vi "TCP Communicator - Active2.vi"() -> ()   [LabVIEW 2019]
panel:
  out "BL_Receive":T1 {"ControlScheme"."Time" format="%<%Y-%m-%d %H:%M:%S>T"; "ControllerConfig"."Time" format="%<%Y-%m-%d %H:%M:%S>T"; "BalancingMotor-All"."BalancingMotor-00"."Time" format="%<%Y-%m-%d %H:%M:%S>T"; "BalancingMotor-All"."BalancingMotor-01"."Time" format="%<%Y-%m-%d %H:%M:%S>T"; "BalancingMotor-All"."BalancingMotor-02"."Time" format="%<%Y-%m-%d %H:%M:%S>T"; "BalancingMotor-All"."BalancingMotor-03"."Time" format="%<%Y-%m-%d %H:%M:%S>T"}
  in  "BL_Send":T1 {"ControlScheme"."Time" format="%<%Y-%m-%d %H:%M:%S>T"; "ControllerConfig"."Time" format="%<%Y-%m-%d %H:%M:%S>T"; "BalancingMotor-All"."BalancingMotor-00"."Time" format="%<%Y-%m-%d %H:%M:%S>T"; "BalancingMotor-All"."BalancingMotor-01"."Time" format="%<%Y-%m-%d %H:%M:%S>T"; "BalancingMotor-All"."BalancingMotor-02"."Time" format="%<%Y-%m-%d %H:%M:%S>T"; "BalancingMotor-All"."BalancingMotor-03"."Time" format="%<%Y-%m-%d %H:%M:%S>T"}
  out "BL_Send2":T1 {"ControlScheme"."Time" format="%<%Y-%m-%d %H:%M:%S>T"; "ControllerConfig"."Time" format="%<%Y-%m-%d %H:%M:%S>T"; "BalancingMotor-All"."BalancingMotor-00"."Time" format="%<%Y-%m-%d %H:%M:%S>T"; "BalancingMotor-All"."BalancingMotor-01"."Time" format="%<%Y-%m-%d %H:%M:%S>T"; "BalancingMotor-All"."BalancingMotor-02"."Time" format="%<%Y-%m-%d %H:%M:%S>T"; "BalancingMotor-All"."BalancingMotor-03"."Time" format="%<%Y-%m-%d %H:%M:%S>T"}
  in  "stop":bool
  in  "Port":u16=6343
  in  "Machine":string="192.168.150.9"
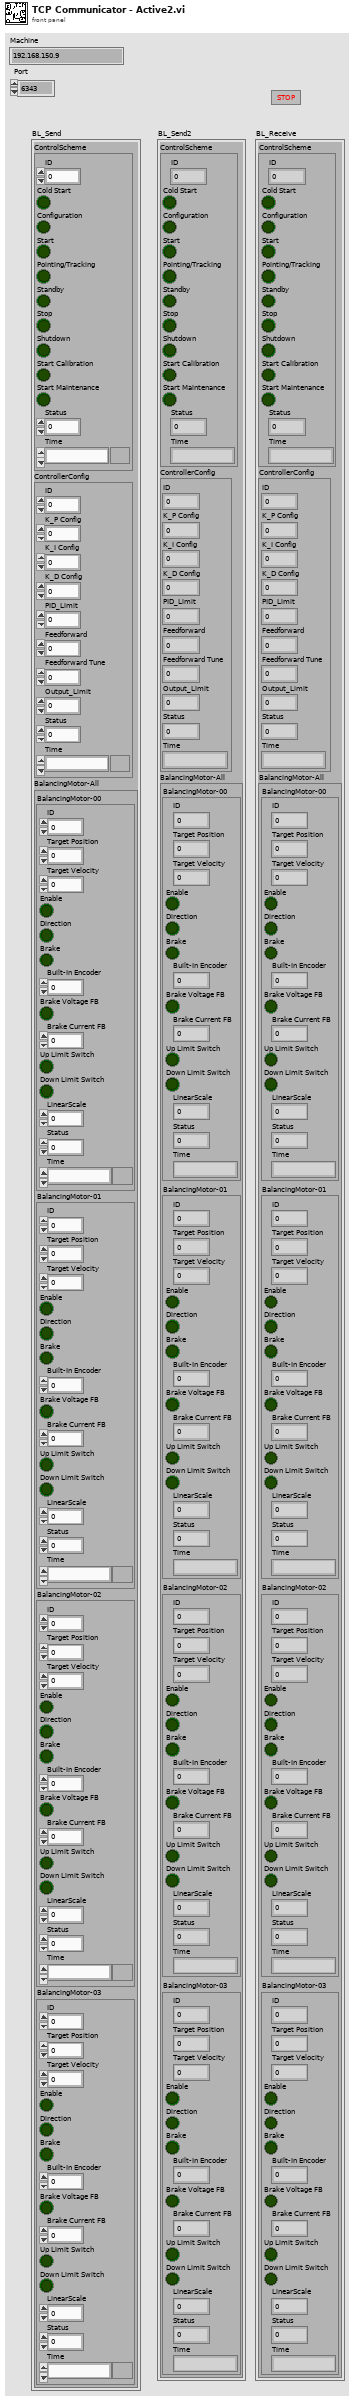
[diagram p1: front panel]
types:
  T1 = cluster{"ControlScheme":cluster{"ID":i32, "Cold Start":bool, "Configuration":bool, "Start":bool, "Pointing/Tracking":bool, "Standby":bool, "Stop":bool, "Shutdown":bool, "Start Calibration":bool, "Start Maintenance":bool, "Status":i16, "Time ":timestamp}, "ControllerConfig":cluster{"ID":i32, "K_P Config":u64, "K_I Config":u64, "K_D Config":u64, "PID_Limit":u64, "Feedforward":u64, "Feedforward Tune":u64, "Output_Limit":u64, "Status":i16, "Time ":timestamp}, "BalancingMotor-All":cluster{"BalancingMotor-00":cluster{"ID":i32, "Target Position":u64, "Target Velocity":u64, "Enable":bool, "Direction":bool, "Brake":bool, "Built-In Encoder":u64, "Brake Voltage FB":bool, "Brake Current FB":u64, "Up Limit Switch":bool, "Down Limit Switch":bool, "LinearScale":u64, "Status":i16, "Time ":timestamp}, "BalancingMotor-01":cluster{"ID":i32, "Target Position":u64, "Target Velocity":u64, "Enable":bool, "Direction":bool, "Brake":bool, "Built-In Encoder":u64, "Brake Voltage FB":bool, "Brake Current FB":u64, "Up Limit Switch":bool, "Down Limit Switch":bool, "LinearScale":u64, "Status":i16, "Time ":timestamp}, "BalancingMotor-02":cluster{"ID":i32, "Target Position":u64, "Target Velocity":u64, "Enable":bool, "Direction":bool, "Brake":bool, "Built-In Encoder":u64, "Brake Voltage FB":bool, "Brake Current FB":u64, "Up Limit Switch":bool, "Down Limit Switch":bool, "LinearScale":u64, "Status":i16, "Time ":timestamp}, "BalancingMotor-03":cluster{"ID":i32, "Target Position":u64, "Target Velocity":u64, "Enable":bool, "Direction":bool, "Brake":bool, "Built-In Encoder":u64, "Brake Voltage FB":bool, "Brake Current FB":u64, "Up Limit Switch":bool, "Down Limit Switch":bool, "LinearScale":u64, "Status":i16, "Time ":timestamp}}}
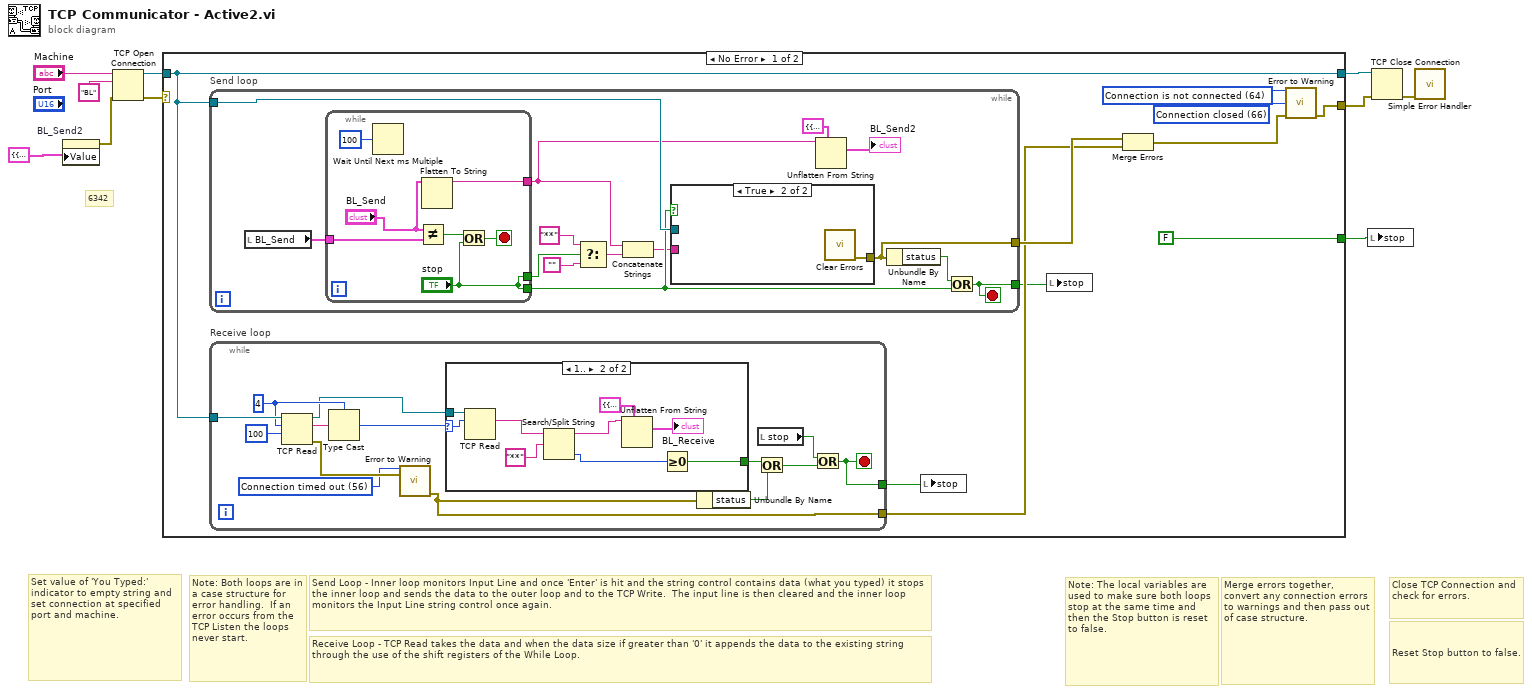
[diagram p0: block diagram]
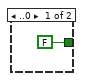
[diagram p2: hidden frame]
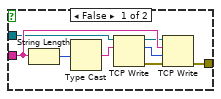
[diagram p3: hidden frame]
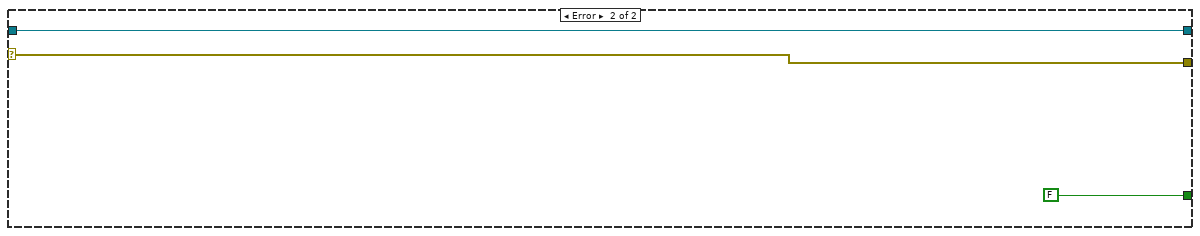
[diagram p4: hidden frame]
diagram:
  # "6342"
  # "Set value of 'You Typed:' indicator to empty string and set connection at specified port and machine."
  # "Send Loop - Inner loop monitors Input Line and once 'Enter' is hit and the string control contains data (what you typed) it stops the inner loop and sends the data to the outer loop and to the TCP Write.  The input line is then cleared and the inner loop monitors the Input Line string control once again."
  # "Receive Loop - TCP Read takes the data and when the data size if greater than '0' it appends the data to the existing string through the use of the shift registers of the While Loop."
  # "Note: The local variables are used to make sure both loops stop at the same time and then the Stop button is reset to false."
  # "Merge errors together, convert any connection errors to warnings and then pass out of case structure."
  # "Note: Both loops are in a case structure for error handling.  If an error occurs from the TCP Listen the loops never start."
  # "Close TCP Connection and check for errors."
  # "Reset Stop button to false."
  n1 = property on="BL_Send2" class="Clust (strict)"("Value"=T1 {"ControlScheme"={"ID"=0, "Cold Start"=FALSE, "Configuration"=FALSE, "Start"=FALSE, "Pointing/Tracking"=FALSE, "Standby"=FALSE, "Stop"=FALSE, "Shutdown"=FALSE, "Start Calibration"=FALSE, "Start Maintenance"=FALSE, "Status"=0, "Time "=timestamp(0 s since 1904-01-01)}, "ControllerConfig"={"ID"=0, "K_P Config"=0, "K_I Config"=0, "K_D Config"=0, "PID_Limit"=0, "Feedforward"=0, "Feedforward Tune"=0, "Output_Limit"=0, "Status"=0, "Time "=timestamp(0 s since 1904-01-01)}, "BalancingMotor-All"={"BalancingMotor-00"={"ID"=0, "Target Position"=0, "Target Velocity"=0, "Enable"=FALSE, "Direction"=FALSE, "Brake"=FALSE, "Built-In Encoder"=0, "Brake Voltage FB"=FALSE, "Brake Current FB"=0, "Up Limit Switch"=FALSE, "Down Limit Switch"=FALSE, "LinearScale"=0, "Status"=0, "Time "=timestamp(0 s since 1904-01-01)}, "BalancingMotor-01"={"ID"=0, "Target Position"=0, "Target Velocity"=0, "Enable"=FALSE, "Direction"=FALSE, "Brake"=FALSE, "Built-In Encoder"=0, "Brake Voltage FB"=FALSE, "Brake Current FB"=0, "Up Limit Switch"=FALSE, "Down Limit Switch"=FALSE, "LinearScale"=0, "Status"=0, "Time "=timestamp(0 s since 1904-01-01)}, "BalancingMotor-02"={"ID"=0, "Target Position"=0, "Target Velocity"=0, "Enable"=FALSE, "Direction"=FALSE, "Brake"=FALSE, "Built-In Encoder"=0, "Brake Voltage FB"=FALSE, "Brake Current FB"=0, "Up Limit Switch"=FALSE, "Down Limit Switch"=FALSE, "LinearScale"=0, "Status"=0, "Time "=timestamp(0 s since 1904-01-01)}, "BalancingMotor-03"={"ID"=0, "Target Position"=0, "Target Velocity"=0, "Enable"=FALSE, "Direction"=FALSE, "Brake"=FALSE, "Built-In Encoder"=0, "Brake Voltage FB"=FALSE, "Brake Current FB"=0, "Up Limit Switch"=FALSE, "Down Limit Switch"=FALSE, "LinearScale"=0, "Status"=0, "Time "=timestamp(0 s since 1904-01-01)}}} ("BL_Send")) -> (error out=w3:errorcluster)  [unwired: 2 in, 1 out]
  n2 = TCP Open Connection(address="Machine", remote port or service name="BL" ("service name"), error in (no error)=w3) -> (connection ID=w8:refnum<k5>, error out=w9:errorcluster)  [unwired: 2 in]
  n3 = case shown="No Error" w9 {
    selector: w9 -> [_ w76]
    tunnel: [w17 w76] -> w6
    tunnel: w8 -> [w11 w77]
    tunnel: [w11 w77] -> w7
    tunnel: [FALSE FALSE] -> w4
    frame No Error {
      w18 = 66 items=["No Error", "Argument Error", "Memory Full", "Out of Zone", "End of File", "File Already Open", "Generic File IO Error", "File Not Found", "File Permission Error", "Disk Full", "Duplicate Path", "Too Many Files Open", "Not Enabled", "Resource File Not Found", "Cannot Add Resource", "Resource Not Found", "Image Not Found", "Image Memory Error", "Pen Does Not Exist", "Config Bad Type", "Config Token Not Found", "Config Parse Error", "Config Memory Error", "Bad External Code Format", "Bad External Code Offset", "External Code Not Present", "Null Window", "Destroy Window Mixup", "Null Menu", "Print Aborted", "Bad Print Record", "Print Driver Error", "Windows Error During Print", "Memory Error During Print", "Print Dialog Error", "Generic Print Error", "Invalid Device Refnum", "Device Not Found", "Device Parameter Error", "Device Unit Error", "Can't Open Device", "Device Call Aborted", "Generic Error", "Cancelled By User", "Object ID Too Low", "Object ID Too High", "Object Not In Heap", "Unknown Heap", "Bad DefProc ID", "DefProc Not In Table", "Message Out Of Range", "Null Method", "Unknown Message", "Manager Call Not Supported", "Bad address", "Connection In progress", "Connection timed out", "Connection is already in progress", "Network attribute not supported", "Network error", "Address in use", "System out of memory", "Connection aborted", "Connection refused", "Connection is not connected", "Connection is already connected", "Connection closed", "Initialize error (interapplication manager)", "Bad occurrence", "Wait on unbound occurrence handler", "Occurrence queue overflow", "Bad path", "Semaphore not signaled", "Unrecognized type (interapplication manager)"] ("3rd Error to Convert")
      w19 = 64 items=["No Error", "Argument Error", "Memory Full", "Out of Zone", "End of File", "File Already Open", "Generic File IO Error", "File Not Found", "File Permission Error", "Disk Full", "Duplicate Path", "Too Many Files Open", "Not Enabled", "Resource File Not Found", "Cannot Add Resource", "Resource Not Found", "Image Not Found", "Image Memory Error", "Pen Does Not Exist", "Config Bad Type", "Config Token Not Found", "Config Parse Error", "Config Memory Error", "Bad External Code Format", "Bad External Code Offset", "External Code Not Present", "Null Window", "Destroy Window Mixup", "Null Menu", "Print Aborted", "Bad Print Record", "Print Driver Error", "Windows Error During Print", "Memory Error During Print", "Print Dialog Error", "Generic Print Error", "Invalid Device Refnum", "Device Not Found", "Device Parameter Error", "Device Unit Error", "Can't Open Device", "Device Call Aborted", "Generic Error", "Cancelled By User", "Object ID Too Low", "Object ID Too High", "Object Not In Heap", "Unknown Heap", "Bad DefProc ID", "DefProc Not In Table", "Message Out Of Range", "Null Method", "Unknown Message", "Manager Call Not Supported", "Bad address", "Connection In progress", "Connection timed out", "Connection is already in progress", "Network attribute not supported", "Network error", "Address in use", "System out of memory", "Connection aborted", "Connection refused", "Connection is not connected", "Connection is already connected", "Connection closed", "Initialize error (interapplication manager)", "Bad occurrence", "Wait on unbound occurrence handler", "Occurrence queue overflow", "Bad path", "Semaphore not signaled", "Unrecognized type (interapplication manager)"] ("1st Error to Convert")
      n4 = while "Send loop" {
        tunnel: w11 -> [w57]
        tunnel: [w58] -> w12
        tunnel: [w53] -> w15
        stop <- w58 stop-if-true
        n5 = local read "BL_Send"() -> (w50:T1)
        n6 = while {
          tunnel: ["stop"] -> w55
          tunnel: ["stop"] -> w51
          tunnel: [w60] -> w49
          tunnel: w50 -> [w62]
          stop <- w63 stop-if-true
          n7 = Wait Until Next ms Multiple(millisecond multiple=u32 100) -> ()  [unwired: 1 out]
          n8 = Not Equal?(x="BL_Send", y=w62) -> (x != y?=w64:bool)
          n9 = Flatten To String(anything="BL_Send") -> (data string=w60:string)  [unwired: 3 in, 2 out]
          n10 = Or(x=w64, y="stop") -> (x .or. y?=w63:bool)
        }
        n11 = Select(t="**", s=w55, f="") -> (s? t:f=w48:string)
        n12 = Concatenate Strings(w49, w48) -> (w47:string)
        n13 = case shown="True" w51 {
          tunnel: w47 -> [w70 _]
          tunnel: [w73 w74] -> w53
          tunnel: w57 -> [w67 _]
          frame False {
            n14 = String Length(string=w70) -> (length=w69:i32)
            n15 = Type Cast(x=w69) -> (*(type *) &x=w68:string)  [unwired: 1 in]
            n16 = TCP Write(connection ID=w67, data in=w68) -> (connection ID out=w66:refnum<k5>, bytes written=w71:i32, error out=w72:errorcluster)  [unwired: 2 in]
            n17 = TCP Write(connection ID=w66, data in=w70, error in (no error)=w72, 9:w71) -> (error out=w73:errorcluster)  [unwired: 2 out]
          }
          frame True {
            n18 = call <vilib>:"Clear Errors.vi"() -> ("error out"=w74:errorcluster)  [unwired: 6 in, 1 out]
          }
        }
        n19 = Unflatten From String(type=T1 {"ControlScheme"={"ID"=0, "Cold Start"=FALSE, "Configuration"=FALSE, "Start"=FALSE, "Pointing/Tracking"=FALSE, "Standby"=FALSE, "Stop"=FALSE, "Shutdown"=FALSE, "Start Calibration"=FALSE, "Start Maintenance"=FALSE, "Status"=0, "Time "=timestamp(0 s since 1904-01-01)}, "ControllerConfig"={"ID"=0, "K_P Config"=0, "K_I Config"=0, "K_D Config"=0, "PID_Limit"=0, "Feedforward"=0, "Feedforward Tune"=0, "Output_Limit"=0, "Status"=0, "Time "=timestamp(0 s since 1904-01-01)}, "BalancingMotor-All"={"BalancingMotor-00"={"ID"=0, "Target Position"=0, "Target Velocity"=0, "Enable"=FALSE, "Direction"=FALSE, "Brake"=FALSE, "Built-In Encoder"=0, "Brake Voltage FB"=FALSE, "Brake Current FB"=0, "Up Limit Switch"=FALSE, "Down Limit Switch"=FALSE, "LinearScale"=0, "Status"=0, "Time "=timestamp(0 s since 1904-01-01)}, "BalancingMotor-01"={"ID"=0, "Target Position"=0, "Target Velocity"=0, "Enable"=FALSE, "Direction"=FALSE, "Brake"=FALSE, "Built-In Encoder"=0, "Brake Voltage FB"=FALSE, "Brake Current FB"=0, "Up Limit Switch"=FALSE, "Down Limit Switch"=FALSE, "LinearScale"=0, "Status"=0, "Time "=timestamp(0 s since 1904-01-01)}, "BalancingMotor-02"={"ID"=0, "Target Position"=0, "Target Velocity"=0, "Enable"=FALSE, "Direction"=FALSE, "Brake"=FALSE, "Built-In Encoder"=0, "Brake Voltage FB"=FALSE, "Brake Current FB"=0, "Up Limit Switch"=FALSE, "Down Limit Switch"=FALSE, "LinearScale"=0, "Status"=0, "Time "=timestamp(0 s since 1904-01-01)}, "BalancingMotor-03"={"ID"=0, "Target Position"=0, "Target Velocity"=0, "Enable"=FALSE, "Direction"=FALSE, "Brake"=FALSE, "Built-In Encoder"=0, "Brake Voltage FB"=FALSE, "Brake Current FB"=0, "Up Limit Switch"=FALSE, "Down Limit Switch"=FALSE, "LinearScale"=0, "Status"=0, "Time "=timestamp(0 s since 1904-01-01)}}} ("BL_Send"), binary string=w49) -> (value=→"BL_Send2":T1)  [unwired: 3 in, 2 out]
        n20 = Unbundle By Name(w53) -> ("status"=w52:bool)
        n21 = Or(x=w52, y=w51) -> (x .or. y?=w58:bool)
      }
      n22 = while "Receive loop" {
        tunnel: [w33] -> w14
        tunnel: [w28] -> w13
        tunnel: w11 -> [w34]
        stop <- w33 stop-if-true
        w23 = 4
        w29 = 56 items=["No Error", "Argument Error", "Memory Full", "Out of Zone", "End of File", "File Already Open", "Generic File IO Error", "File Not Found", "File Permission Error", "Disk Full", "Duplicate Path", "Too Many Files Open", "Not Enabled", "Resource File Not Found", "Cannot Add Resource", "Resource Not Found", "Image Not Found", "Image Memory Error", "Pen Does Not Exist", "Config Bad Type", "Config Token Not Found", "Config Parse Error", "Config Memory Error", "Bad External Code Format", "Bad External Code Offset", "External Code Not Present", "Null Window", "Destroy Window Mixup", "Null Menu", "Print Aborted", "Bad Print Record", "Print Driver Error", "Windows Error During Print", "Memory Error During Print", "Print Dialog Error", "Generic Print Error", "Invalid Device Refnum", "Device Not Found", "Device Parameter Error", "Device Unit Error", "Can't Open Device", "Device Call Aborted", "Generic Error", "Cancelled By User", "Object ID Too Low", "Object ID Too High", "Object Not In Heap", "Unknown Heap", "Bad DefProc ID", "DefProc Not In Table", "Message Out Of Range", "Null Method", "Unknown Message", "Manager Call Not Supported", "Bad address", "Connection In progress", "Connection timed out", "Connection is already in progress", "Network attribute not supported", "Network error", "Address in use", "System out of memory", "Connection aborted", "Connection refused", "Connection is not connected", "Connection is already connected", "Connection closed", "Initialize error (interapplication manager)", "Bad occurrence", "Wait on unbound occurrence handler", "Occurrence queue overflow", "Bad path", "Semaphore not signaled", "Unrecognized type (interapplication manager)"] ("1st Error to Convert")
        n23 = TCP Read(connection ID=w34, bytes to read=w23, 9:100) -> (connection ID out=w21:refnum<k5>, data out=w24:string, error out=w30:errorcluster)  [unwired: 2 in]
        n24 = Type Cast(type=w23, x=w24) -> (*(type *) &x=w22:i32)
        n25 = call <vilib>:"Error to Warning.vi"("1st Error to Convert"=w29, "error in"=w30) -> ("warning out"=w28:errorcluster)  [unwired: 13 in]
        n26 = case shown="1.." w22 {
          selector: w22 -> [_ w44]
          tunnel: [FALSE w40] -> w32
          tunnel: w21 -> [_ w43]
          frame ..0 {
          }
          frame 1.. {
            n27 = TCP Read(connection ID=w43, bytes to read=w44) -> (data out=w37:string)  [unwired: 3 in, 2 out]
            n28 = Search/Split String(string=w37, search string/char (-)="**") -> (substring before match=w36:string, offset of match=w42:i32)  [unwired: 1 in, 1 out]
            n29 = Unflatten From String(type=T1 {"ControlScheme"={"ID"=0, "Cold Start"=FALSE, "Configuration"=FALSE, "Start"=FALSE, "Pointing/Tracking"=FALSE, "Standby"=FALSE, "Stop"=FALSE, "Shutdown"=FALSE, "Start Calibration"=FALSE, "Start Maintenance"=FALSE, "Status"=0, "Time "=timestamp(0 s since 1904-01-01)}, "ControllerConfig"={"ID"=0, "K_P Config"=0, "K_I Config"=0, "K_D Config"=0, "PID_Limit"=0, "Feedforward"=0, "Feedforward Tune"=0, "Output_Limit"=0, "Status"=0, "Time "=timestamp(0 s since 1904-01-01)}, "BalancingMotor-All"={"BalancingMotor-00"={"ID"=0, "Target Position"=0, "Target Velocity"=0, "Enable"=FALSE, "Direction"=FALSE, "Brake"=FALSE, "Built-In Encoder"=0, "Brake Voltage FB"=FALSE, "Brake Current FB"=0, "Up Limit Switch"=FALSE, "Down Limit Switch"=FALSE, "LinearScale"=0, "Status"=0, "Time "=timestamp(0 s since 1904-01-01)}, "BalancingMotor-01"={"ID"=0, "Target Position"=0, "Target Velocity"=0, "Enable"=FALSE, "Direction"=FALSE, "Brake"=FALSE, "Built-In Encoder"=0, "Brake Voltage FB"=FALSE, "Brake Current FB"=0, "Up Limit Switch"=FALSE, "Down Limit Switch"=FALSE, "LinearScale"=0, "Status"=0, "Time "=timestamp(0 s since 1904-01-01)}, "BalancingMotor-02"={"ID"=0, "Target Position"=0, "Target Velocity"=0, "Enable"=FALSE, "Direction"=FALSE, "Brake"=FALSE, "Built-In Encoder"=0, "Brake Voltage FB"=FALSE, "Brake Current FB"=0, "Up Limit Switch"=FALSE, "Down Limit Switch"=FALSE, "LinearScale"=0, "Status"=0, "Time "=timestamp(0 s since 1904-01-01)}, "BalancingMotor-03"={"ID"=0, "Target Position"=0, "Target Velocity"=0, "Enable"=FALSE, "Direction"=FALSE, "Brake"=FALSE, "Built-In Encoder"=0, "Brake Voltage FB"=FALSE, "Brake Current FB"=0, "Up Limit Switch"=FALSE, "Down Limit Switch"=FALSE, "LinearScale"=0, "Status"=0, "Time "=timestamp(0 s since 1904-01-01)}}} ("BL_Send"), binary string=w36) -> (value=→"BL_Receive":T1)  [unwired: 3 in, 2 out]
            n30 = Greater Or Equal To 0?(x=w42) -> (x >= 0?=w40:bool)
          }
        }
        n31 = Unbundle By Name(w28) -> ("status"=w27:bool)
        n32 = Or(x=w32, y=w27) -> (x .or. y?=w25:bool)
        n33 = local read "stop"() -> (w26:bool)
        n34 = Or(x=w26, y=w25) -> (x .or. y?=w33:bool)
      }
      n35 = local write "stop"(w14) -> ()
      n36 = local write "stop"(w12) -> ()
      n37 = Merge Errors(w15, w13) -> (w20:errorcluster)
      n38 = call <vilib>:"Error to Warning.vi"("1st Error to Convert"=w19, "3rd Error to Convert"=w18, "error in"=w20) -> ("warning out"=w17:errorcluster)  [unwired: 12 in]
    }
    frame Error {
    }
  }
  n39 = local write "stop"(w4) -> ()
  n40 = TCP Close Connection(connection ID=w7, error in (no error)=w6) -> (error out=w5:errorcluster)  [unwired: 1 in, 1 out]
  n41 = call <vilib>:"Simple Error Handler.vi"("error in (no error)"=w5) -> ()  [unwired: 4 in, 5 out]
